vi "Producer.vi"(8 "Error In":errorcluster, 11 "App Data In":T2={"Console log"="", "GUI_Events"={"To_GUI-Producer"=refnum, "To_GUI-Error_message"=refnum, "To_GUI-msg_list"=refnum, "To_GUI-Session"=refnum, "To_GUI-Pre-Session"=refnum, "To_GUI-Consumer"=refnum}, "Function_Queue"={"Queue_MIDI_Handler"=refnum, "Queue_Session"=refnum, "Queue_Producer"=refnum, "Queue_Consumer"=refnum}, "Timout-Time[ms]"=0, "MIDI-Messages"=[], "Com Session State"=enum."Active Session", "Result Data"={"Diff"=[], "Tx Byte"=[], "Rx Byte"=[], "Send Log"=[], "Parsed Data"={"Tx MIDI Tag"=[], "Tx MIDI Parsed Data"=[], "Tx Error"=[], "Tx Running States"=[], "Rx MIDI Tag"=[], "Rx MIDI Parsed Data"=[], "Rx Error"=[], "Rx Running States"=[], "Diff"=[]}}, "Get #"=[], "CPU(ms)"=0}) -> (0 "Error Out":errorcluster, 3 "Producer-Data":T11={"Queue_Producer"=refnum, "Queue_Consumer"=refnum, "To_GUI-Error_message"=refnum, "Rx-Data"=[], "Tx-Data"=[], "Console log"="", "Communication Settings"={"Tx Protocol"=enum."Not Active", "Rx Protocol"=enum."Serial", "Serial"={"Tx Port"="", "Rx Port"="", "Baud rate"=31250, "Parity"=enum."Space", "Data bits"=8, "Stop bits"=10, "Flow control"=enum."None", "Tx Resource"="", "Rx Resource"=""}, "MIDI Device"={"Input uDevice ID"=0, "Output uDevice ID"=0, "hmidiout Handle"=0, "hmidiin Handle"=0}, "Bluetooth"={"Dummy"=""}, "USB"={"Dummy"=""}}, "MIDI-Messages"=[], "Queue_Session"=refnum, "To_GUI-Pre-Session"=refnum, "To_GUI-Producer"=refnum, "Tx Info"={"Datatype"=[], "Bytesize"=[], "Strings"=[], "ByteSum"=0}, "Payload"=variant, "Timout-Time[ms]"=0, "To_GUI-Session"=refnum, "CPU(ms)"=0})   [LabVIEW 2019]
doc: "This VI send and receive data to nRF."
uses:
  Common/Controls/Application_Data.ctl
  Common/Controls/App_Events.ctl
  Common/Controls/App_Queues.ctl
  Common/Controls/Application_Message.ctl
  Common/Controls/Application_State.ctl
  MIDI/Controls/MIDI-Message_Array.ctl
  MIDI/Controls/MIDI-Message_Cluster.ctl
  MIDI/Controls/Meta_Commands.ctl
  Controls/Session_State.ctl
  Consumer/Controls/Consumer_Result.ctl
  Consumer/Controls/Parsed_Data.ctl
  Controls/Producer-Data.ctl
  Common/Controls/Communication_Settings.ctl
  Common/Controls/Communication_Protocols.ctl
  Controls/Prod - Tx_Info.ctl
  <vilib>/Utility/error.llb/DialogType.ctl
panel:
  in  "Control Tab":T1(tab)
  out "Log":string
  out "Error Message":string
  out "VI-filename":string
  out "VI Path":path
  out "Code Size":u32
  out "Revision Number":u32
  in  "Tool Bar:Visible":bool
  in  "Execution:Show Front Panel On Call":bool
  out "VI-Name":string
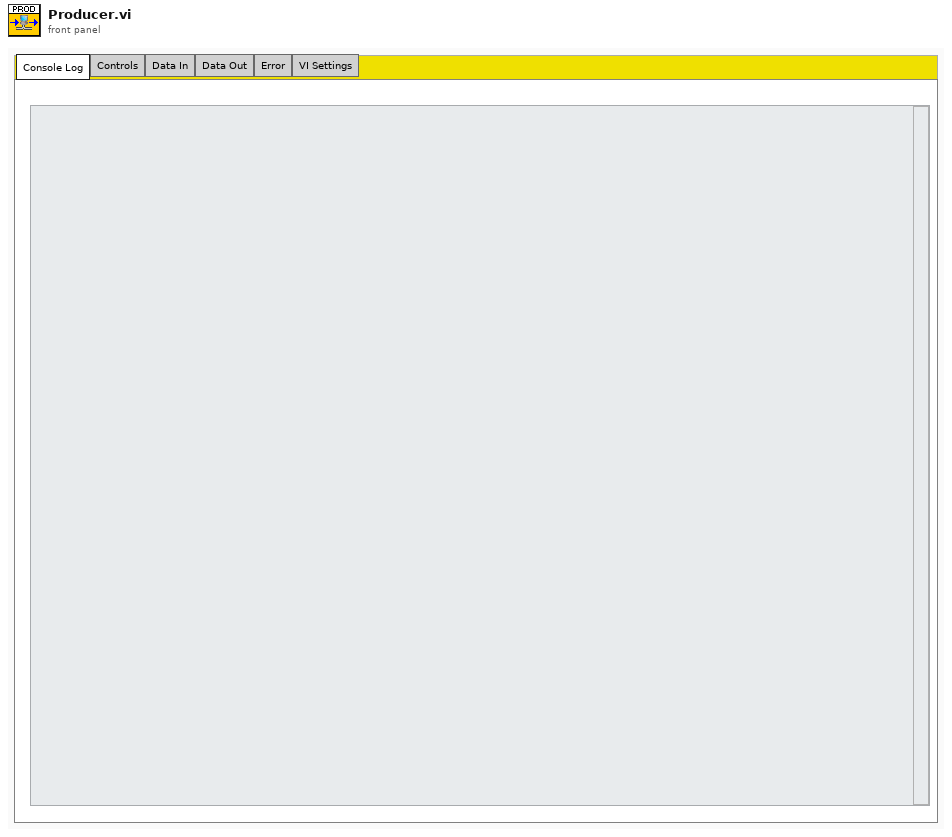
[diagram p1: front panel]
types:
  T1 = enum32{"Console Log", "Controls", "Data In", "Data Out", "Error", "VI Settings"}
  T2 = typedef "Application_Data.ctl" = cluster{"Console log":string, "GUI_Events":T3, "Function_Queue":T4, "Timout-Time[ms]":i32, "MIDI-Messages":T5, "Com Session State":T8, "Result Data":T9, "Get #":bool[], "CPU(ms)":u32}
  T3 = typedef "App_Events.ctl" = cluster{"To_GUI-Producer":refnum<user-event>, "To_GUI-Error_message":refnum<user-event>, "To_GUI-msg_list":refnum<user-event>, "To_GUI-Session":refnum<user-event>, "To_GUI-Pre-Session":refnum<user-event>, "To_GUI-Consumer":refnum<user-event>}
  T4 = typedef "App_Queues.ctl" = cluster{"Queue_MIDI_Handler":refnum<queue>, "Queue_Session":refnum<queue>, "Queue_Producer":refnum<queue>, "Queue_Consumer":refnum<queue>}
  T5 = typedef "MIDI-Message_Array.ctl" = T6[]
  T6 = typedef "MIDI-Message_Cluster.ctl" = cluster{"Message Name":string, "Meta value":i32, "Datastring":string, "Datatype":T7}
  T7 = typedef "Meta_Commands.ctl" = enum16{"No Data", "Pause", "Loop", "Wait for Rx", "Delay", "Break", "MIDI"}
  T8 = typedef "Session_State.ctl" = enum16{"Wait to begin", "Active Session", "Pause", "Wait for Response", "Stop", "Restart", "Inspect", "Exit"}
  T9 = typedef "Consumer_Result.ctl" = cluster{"Diff":bool[], "Tx Byte":string[], "Rx Byte":string[], "Send Log":string[], "Parsed Data":T10}
  T10 = typedef "Parsed_Data.ctl" = cluster{"Tx MIDI Tag":string[], "Tx MIDI Parsed Data":string[], "Tx Error":bool[], "Tx Running States":string[], "Rx MIDI Tag":string[], "Rx MIDI Parsed Data":string[], "Rx Error":bool[], "Rx Running States":string[], "Diff":bool[]}
  T11 = typedef "Producer-Data.ctl" = cluster{"Queue_Producer":refnum<queue>, "Queue_Consumer":refnum<queue>, "To_GUI-Error_message":refnum<user-event>, "Rx-Data":i8[], "Tx-Data":i8[], "Console log":string, "Communication Settings":T12, "MIDI-Messages":T5, "Queue_Session":refnum<queue>, "To_GUI-Pre-Session":refnum<user-event>, "To_GUI-Producer":refnum<user-event>, "Tx Info":T14, "Payload":variant, "Timout-Time[ms]":i32, "To_GUI-Session":refnum<user-event>, "CPU(ms)":u32}
  T12 = typedef "Communication_Settings.ctl" = cluster{"Tx Protocol":T13, "Rx Protocol":T13, "Serial":cluster{"Tx Port":refnum<visa-resource-name>, "Rx Port":refnum<visa-resource-name>, "Baud rate":i32, "Parity":enum16{"None", "Odd", "Even", "Mark", "Space"}, "Data bits":i32, "Stop bits":i32, "Flow control":enum16{"None", "XON/XOFF", "RTS/CTS", "XON/XOFF & RTS/CTS", "DTR/DSR", "XON/XOFF & DTR/DSR"}, "Tx Resource":refnum<visa-resource-name>, "Rx Resource":refnum<visa-resource-name>}, "MIDI Device":cluster{"Input uDevice ID":u32, "Output uDevice ID":u32, "hmidiout Handle":i32, "hmidiin Handle":i32}, "Bluetooth":cluster{"Dummy":string}, "USB":cluster{"Dummy":string}}
  T13 = typedef "Communication_Protocols.ctl" = enum16{"Serial", "Bluetooth", "USB-MIDI", "MIDI (Audio Device)", "Not Active"}
  T14 = typedef "Prod - Tx_Info.ctl" = cluster{"Datatype":T7[], "Bytesize":i32[], "Strings":string[], "ByteSum":i32}
  T15 = typedef "Application_State.ctl" = enum16{"Idle", "Initiate", "MH Load Messages", "Prepare for Tx", "Settings", "Com Session", "Receive", "Data", "Uninitialize", "Quit Message", "Export Send"}
  T16 = typedef "DialogType.ctl" = u16
  T17 = typedef "Application_Message.ctl" = cluster{"Application State":T15, "Payload":variant}
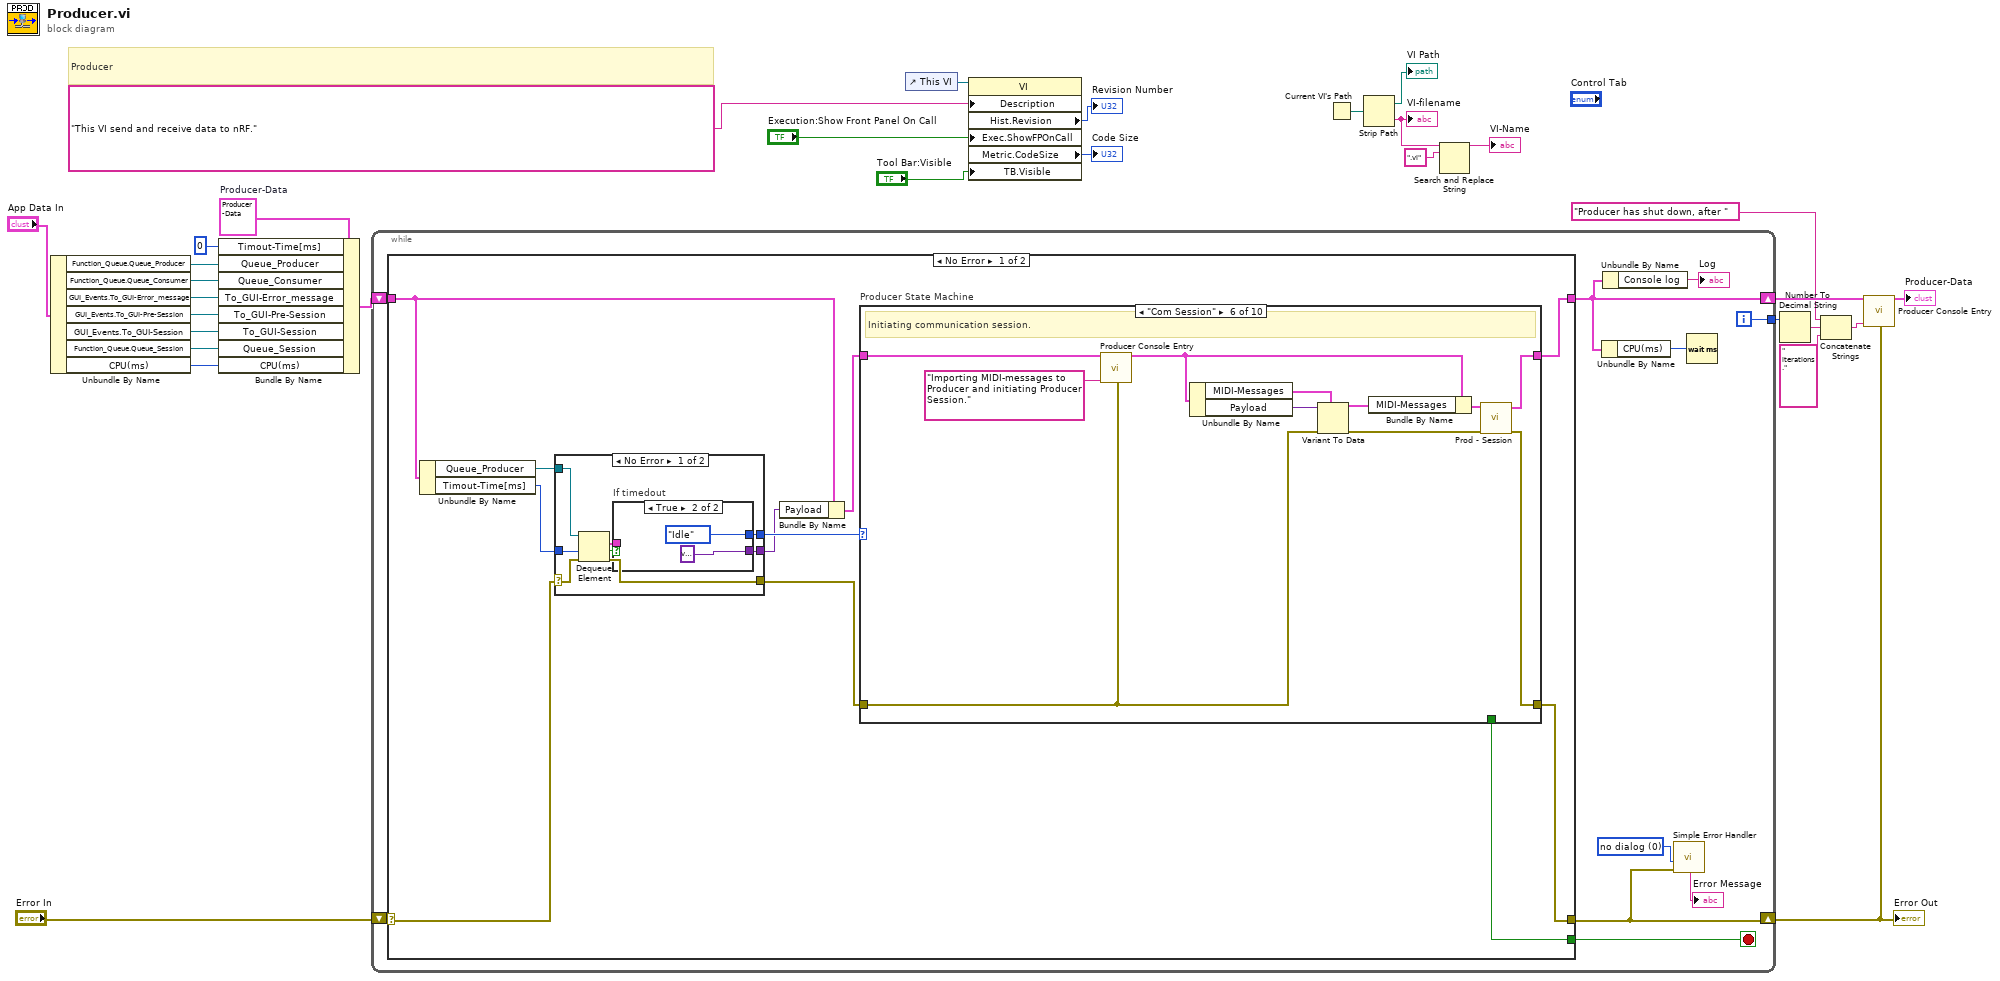
[diagram p0: block diagram]
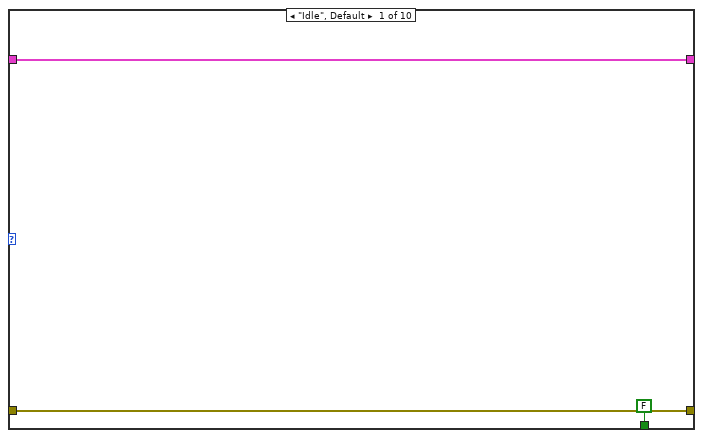
[diagram p2: hidden frame]
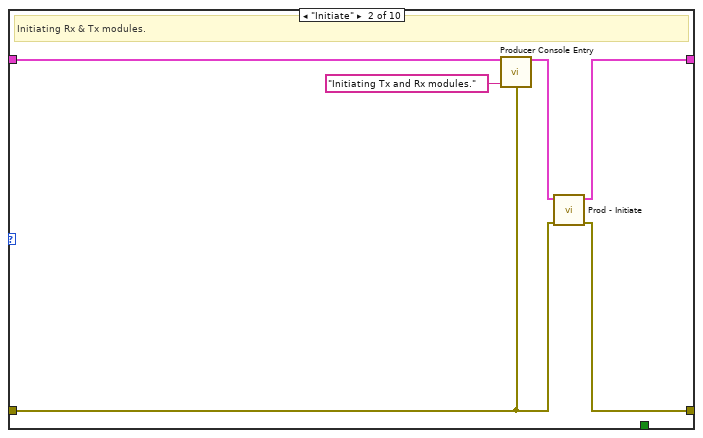
[diagram p3: hidden frame]
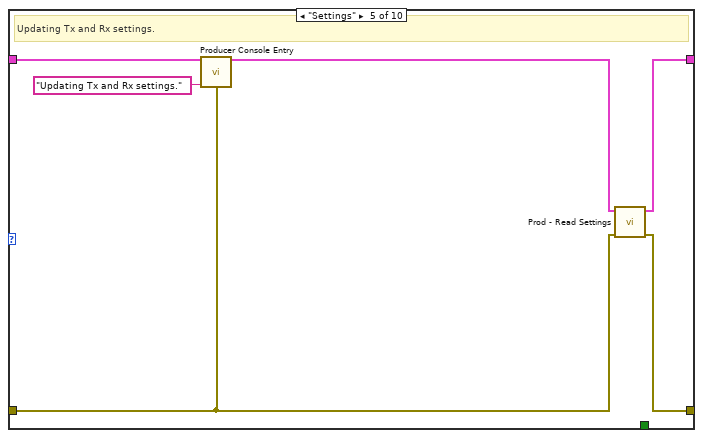
[diagram p6: hidden frame]
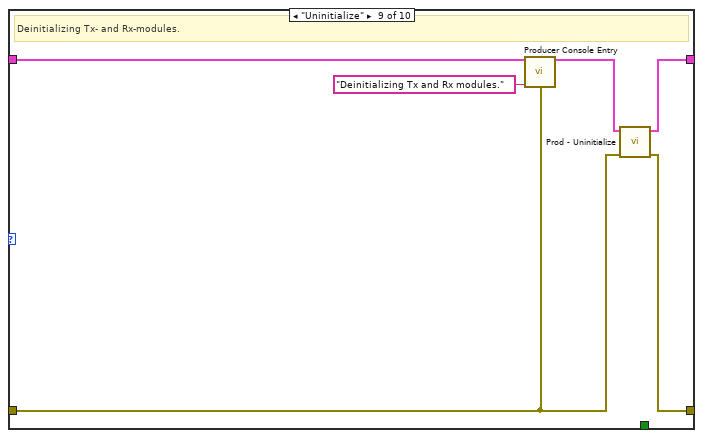
[diagram p9: hidden frame]
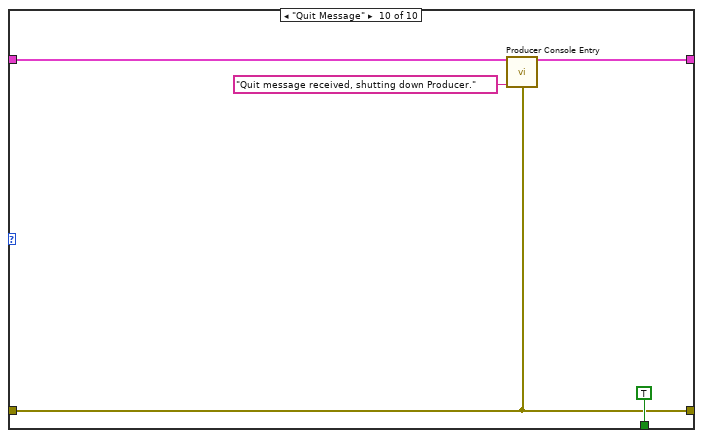
[diagram p10: hidden frame]
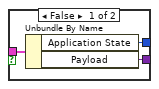
[diagram p11: hidden frame]
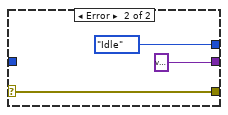
[diagram p12: hidden frame]
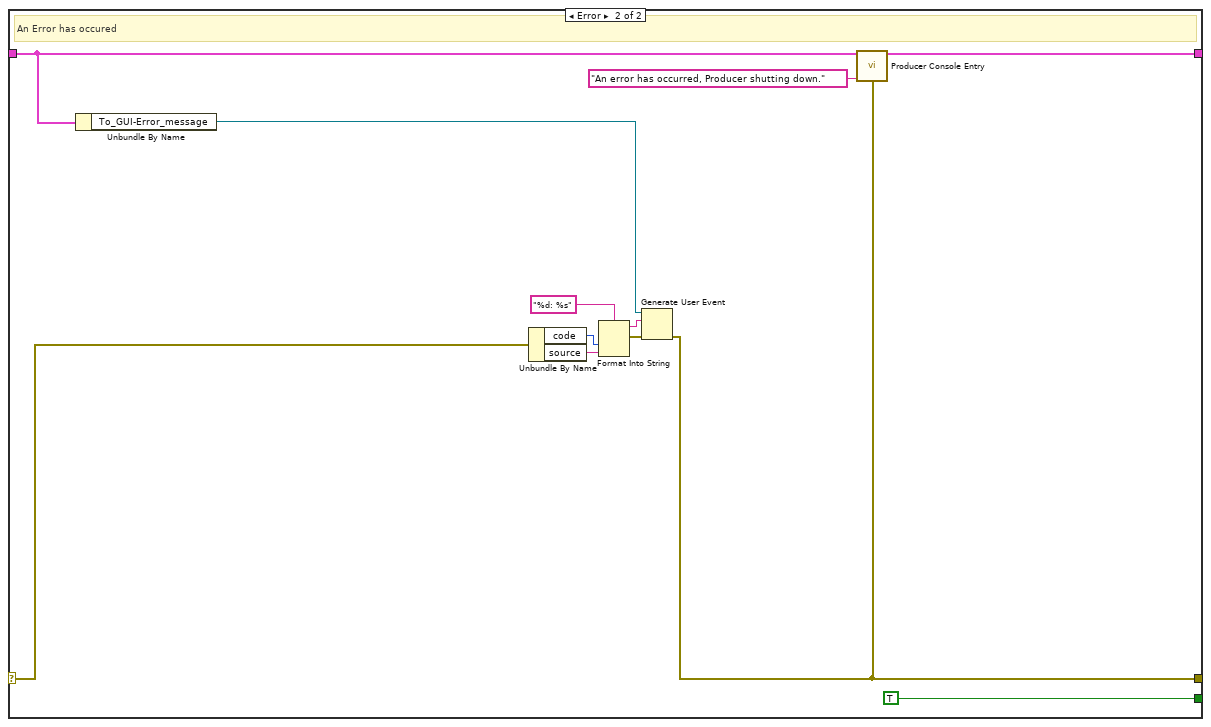
[diagram p13: hidden frame]
diagram:
  w16 = T11 {"Queue_Producer"=refnum, "Queue_Consumer"=refnum, "To_GUI-Error_message"=refnum, "Rx-Data"=[], "Tx-Data"=[], "Console log"="", "Communication Settings"={"Tx Protocol"=enum."Serial", "Rx Protocol"=enum."Serial", "Serial"={"Tx Port"="", "Rx Port"="", "Baud rate"=31250, "Parity"=enum."None", "Data bits"=8, "Stop bits"=10, "Flow control"=enum."None", "Tx Resource"="", "Rx Resource"=""}, "MIDI Device"={"Input uDevice ID"=0, "Output uDevice ID"=0, "hmidiout Handle"=0, "hmidiin Handle"=0}, "Bluetooth"={"Dummy"=""}, "USB"={"Dummy"=""}}, "MIDI-Messages"=[], "Queue_Session"=refnum, "To_GUI-Pre-Session"=refnum, "To_GUI-Producer"=refnum, "Tx Info"={"Datatype"=[], "Bytesize"=[], "Strings"=[], "ByteSum"=0}, "Payload"=variant, "Timout-Time[ms]"=0, "To_GUI-Session"=refnum, "CPU(ms)"=0}  # Producer-Data
  # "Producer"
  n1 = Unbundle By Name("App Data In") -> ("Function_Queue.Queue_Producer"=w14:refnum<queue>, "Function_Queue.Queue_Consumer"=w13:refnum<queue>, "GUI_Events.To_GUI-Error_message"=w19:refnum<user-event>, "GUI_Events.To_GUI-Pre-Session"=w15:refnum<user-event>, "GUI_Events.To_GUI-Session"=w10:refnum<user-event>, "Function_Queue.Queue_Session"=w11:refnum<queue>, "CPU(ms)"=w1:u32)
  n2 = Bundle By Name(cluster=w16, "Timout-Time[ms]"=0, "Queue_Producer"=w14, "Queue_Consumer"=w13, "To_GUI-Error_message"=w19, "To_GUI-Pre-Session"=w15, "To_GUI-Session"=w10, "Queue_Session"=w11, "CPU(ms)"=w1) -> (w18:T11)
  n3 = while {
    shift-right: [w37] -> w7
    shift-left: "Error In" -> [w41]
    shift-right: [w33] -> w8
    shift-left: w18 -> [w39]
    tunnel: [w34] -> w3
    i -> [w34]
    stop <- w40 stop-if-true
    w36 = T16 0 items=["no dialog", "OK message", "continue or stop message", "OK message + warnings", "continue/stop + warnings"] ("type of dialog (OK msg:1)")
    n4 = case shown="No Error" w41 {
      selector: w41 -> [w50 w115]
      tunnel: [w43 w114] -> w37
      tunnel: [w42 TRUE] -> w40
      tunnel: w39 -> [w48 w117]
      tunnel: [w45 w118] -> w33
      frame No Error {
        n5 = Unbundle By Name(w48) -> ("Queue_Producer"=w52:refnum<queue>, "Timout-Time[ms]"=w51:i32)
        n6 = case shown="No Error" w50 {
          selector: w50 -> [w102 w113]
          tunnel: [w101 w113] -> w44
          tunnel: [w104 Application_State."Idle" ("Data_Type")] -> w49
          tunnel: [w103 variant ("Payload")] -> w47
          tunnel: w52 -> [w100 _]
          tunnel: w51 -> [w99 _]
          frame No Error {
            n7 = Dequeue Element(queue=w100, timeout in ms (-1)=w99, error in (no error)=w102) -> (element=w105:T17, timed out?=w98:bool, error out=w101:errorcluster)  [unwired: 1 out]
            n8 = case "If timedout" shown="True" w98 {
              tunnel: w105 -> [w108 _]
              tunnel: [w107 Application_State."Idle" ("Data_Type")] -> w104
              tunnel: [w106 variant ("Payload")] -> w103
              frame False {
                n9 = Unbundle By Name(w108) -> ("Application State"=w107:T15, "Payload"=w106:variant)
              }
              frame True {
              }
            }
          }
          frame Error {
          }
        }
        n10 = Bundle By Name(cluster=w48, "Payload"=w47) -> (w46:T11)
        n11 = case "Producer State Machine" shown="\"Com Session\"" w49 {
          tunnel: w46 -> [w55 w59 w63 w65 w69 w74 w83 w86 w90 w96]
          tunnel: [w55 w56 w63 w65 w71 w76 w83 w86 w92 w95] -> w45
          tunnel: w44 -> [w54 w58 w62 w64 w67 w73 w84 w85 w88 w93]
          tunnel: [w54 w60 w62 w64 w70 w77 w84 w85 w91 w93] -> w43
          tunnel: [FALSE _ _ _ _ _ _ _ _ TRUE] -> w42
          frame "Idle", Default {
          }
          frame "Initiate" {
            # "Initiating Rx & Tx modules."
            n12 = call "Producer Console Entry.vi"("Prod-Data In"=w59, "Console Entry"="Initiating Tx and Rx modules.", "Error In"=w58) -> ("Prod-Data Out"=w57:T11)  [unwired: 12 in]
            n13 = call "Prod - Initiate.vi"("Error In"=w58, "Prod-Data In"=w57) -> ("Error Out"=w60:errorcluster, "Prod-Data Out"=w56:T11)  [unwired: 8 in]
          }
          frame "MH Load Messages" {
          }
          frame "Prepare for Tx" {
          }
          frame "Settings" {
            # "Updating Tx and Rx settings."
            n14 = call "Producer Console Entry.vi"("Prod-Data In"=w69, "Console Entry"="Updating Tx and Rx settings.", "Error In"=w67) -> ("Prod-Data Out"=w68:T11)  [unwired: 12 in]
            n15 = call "Prod - Read Settings.vi"("Error In"=w67, "Prod Data In"=w68) -> ("Error Out"=w70:errorcluster, "Prod Data Out"=w71:T11)  [unwired: 8 in]
          }
          frame "Com Session" {
            # "Initiating communication session."
            n16 = call "Producer Console Entry.vi"("Prod-Data In"=w74, "Console Entry"="Importing MIDI-messages to Producer and initiating Producer Session.", "Error In"=w73) -> ("Prod-Data Out"=w75:T11)  [unwired: 12 in]
            n17 = Unbundle By Name(w75) -> ("MIDI-Messages"=w81:T5, "Payload"=w82:variant)
            n18 = Variant To Data(error in=w73, type=w81, Variant=w82) -> (data=w79:T5, error out=w80:errorcluster)
            n19 = Bundle By Name(cluster=w75, "MIDI-Messages"=w79) -> (w78:T11)
            n20 = call "Prod - Session.vi"("Error In"=w80, "Prod-Data In"=w78) -> ("Error Out"=w77:errorcluster, "Prod-Data Out"=w76:T11)  [unwired: 8 in]
          }
          frame "Receive" {
          }
          frame "Data" {
          }
          frame "Uninitialize" {
            # "Deinitializing Tx- and Rx-modules."
            n21 = call "Producer Console Entry.vi"("Prod-Data In"=w90, "Console Entry"="Deinitializing Tx and Rx modules.", "Error In"=w88) -> ("Prod-Data Out"=w89:T11)  [unwired: 12 in]
            n22 = call "Prod - Uninitialize.vi"("Error In"=w88, "Prod-Data In"=w89) -> ("Error Out"=w91:errorcluster, "Prod-Data Out"=w92:T11)  [unwired: 8 in]
          }
          frame "Quit Message" {
            n23 = call "Producer Console Entry.vi"("Prod-Data In"=w96, "Console Entry"="Quit message received, shutting down Producer.", "Error In"=w93) -> ("Prod-Data Out"=w95:T11)  [unwired: 12 in]
          }
        }
      }
      frame Error {
        # "An Error has occured"
        n24 = Unbundle By Name(w117) -> ("To_GUI-Error_message"=w119:refnum<user-event>)
        n25 = Unbundle By Name(w115) -> ("code"=w124:i32, "source"=w123:string)
        n26 = Format Into String(format string="%d: %s", w124, w123) -> (resulting string=w122:string, error out=w120:errorcluster)  [unwired: 2 in]
        n27 = Generate User Event(user event=w119, event data cluster=w122, error in=w120) -> (error out=w114:errorcluster)  [unwired: 1 in, 1 out]
        n28 = call "Producer Console Entry.vi"("Prod-Data In"=w117, "Console Entry"="An error has occurred, Producer shutting down.", "Error In"=w114) -> ("Prod-Data Out"=w118:T11)  [unwired: 12 in]
      }
    }
    n29 = Unbundle By Name(w33) -> ("CPU(ms)"=w32:u32)
    n30 = Unbundle By Name(w33) -> ("Console log"=→"Log":string)
    n31 = call <vilib>:"Simple Error Handler.vi"("type of dialog (OK msg:1)"=w36, "error in (no error)"=w37) -> ("message"=→"Error Message":string)  [unwired: 3 in, 4 out]
    n32 = Wait (ms)(milliseconds to wait=w32) -> ()  [unwired: 1 out]
  }
  "Error Out" <- w7
  n33 = control-ref of="This VI"() -> (w25:refnum<vi>)
  n34 = property class="VI"(reference=w25, "Description"="This VI send and receive data to nRF.", "Exec.ShowFPOnCall"="Execution:Show Front Panel On Call", "TB.Visible"="Tool Bar:Visible") -> ("Hist.Revision"=→"Revision Number":u32, "Metric.CodeSize"=→"Code Size":u32)  [unwired: 1 in, 2 out]
  n35 = Current VI's Path() -> (path=w31:path)
  n36 = Strip Path(path=w31) -> (stripped path=→"VI Path":path, name=w22:string)
  "VI-filename" <- w22
  n37 = Search and Replace String(input string=w22, search string=".vi") -> (result string=→"VI-Name":string)  [unwired: 6 in, 3 out]
  n38 = Number To Decimal String(number=w3) -> (decimal integer string=w4:string)  [unwired: 1 in]
  n39 = Concatenate Strings("Producer has shut down, after " ("Console Entry"), w4, " iterations." ("string")) -> (w6:string)
  n40 = call "Producer Console Entry.vi"("Prod-Data In"=w8, "Console Entry"=w6, "Error In"=w7) -> ("Prod-Data Out"=→"Producer-Data":T11)  [unwired: 12 in]
